vi "write_ini_SavedPos.vi"(8 "error in (no error)":errorcluster caption="错误输入（无错误）", 10 "file ref in":T1, 11 "MotorSystem 输入":refnum<class "MotorSystem.lvclass">) -> (0 "error out":errorcluster caption="错误输出", 2 "file ref out":T1, 3 "MotorSystem 输出":refnum<class "MotorSystem.lvclass">)   [LabVIEW 2016, in "MotionControl_UFO_3DOF.lvlib" / "MotorSystem.lvclass"]
uses:
  <userlib>/MotionControl_UFO_3DOF/MotorSystem/MotorSystem.lvclass
  <vilib>/Utility/config.llb/Config Data RefNum.ctl
  <userlib>/MotionControl_UFO_3DOF/MotorSystem/MotorSystem.lvclass/MotorSystem.ctl
  <vilib>/Utility/config.llb/Write Key (I32).vi
  <vilib>/Utility/config.llb/Write Key (String).vi
  <vilib>/Utility/config.llb/Write Key (Double).vi
  <vilib>/Utility/config.llb/NI_LVConfig.lvlib
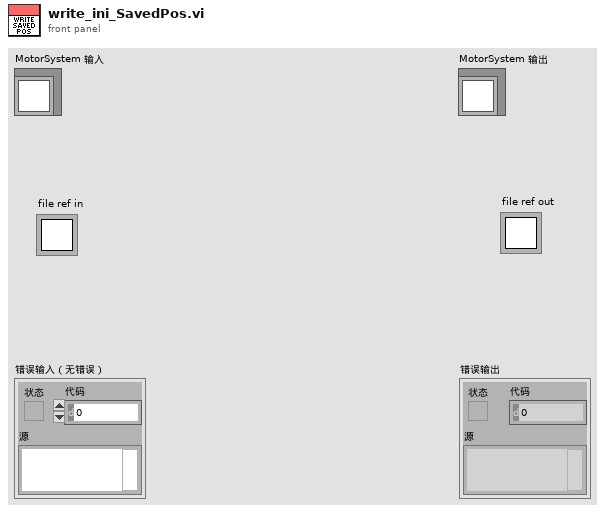
[diagram p1: front panel]
types:
  T1 = typedef "NI_LVConfig.lvlib/Config Data RefNum.ctl" = refnum<k1>
  T2 = typedef "MotionControl_UFO_3DOF.lvlib/MotorSystem.lvclass/SavedPosCluster.ctl" = cluster{"name":string, "command list":T3}
  T3 = typedef "MotionControl_UFO_3DOF.lvlib/MotorSystem.lvclass/CommandList.ctl" = cluster{"cmd":T4, "cmd info":T5[]}[]
  T4 = typedef "MotionControl_UFO_3DOF.lvlib/MotorSystem.lvclass/cmd_system.ctl" = enum16{"NONE", "MOVE_SYSTEM", "WAIT_UNTIL_MOVE_DONE", "EXIT", "WAIT_UNTIL_SELECTED_MOVE_DONE", "WAIT_A_TIME"}
  T5 = typedef "MotionControl_UFO_3DOF.lvlib/MotorSystem.lvclass/SavedDimensionCluster.ctl" = cluster{"dimension name":string, "pos":dbl, "unit mode":T6, "unit conversion ratio":dbl}
  T6 = typedef "MotionControl_UFO_3DOF.lvlib/OneMotion.lvclass/unit mode.ctl" = enum16{"motor (pulse)", "linear (mm) or radial (degree)"}
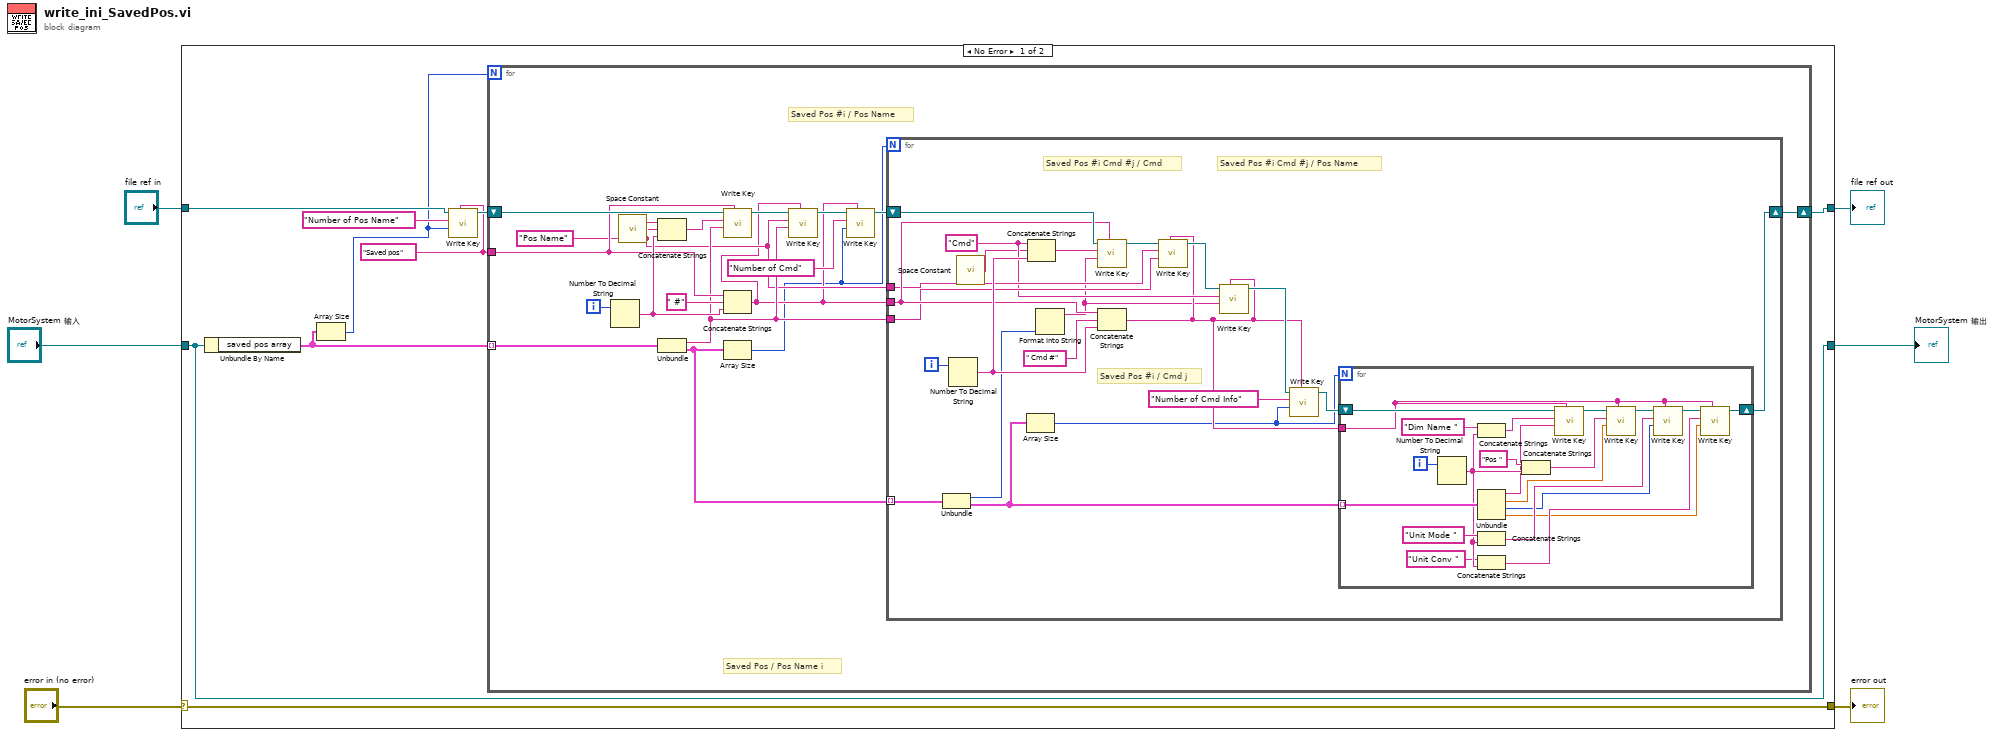
[diagram p0: block diagram]
diagram:
  n1 = case shown="No Error" "error in (no error)" {
    selector: "error in (no error)" -> [w15 w79]
    tunnel: [w15 w79] -> w5
    tunnel: [w14 w78] -> w3
    tunnel: "MotorSystem 输入" -> [w14 w78]
    tunnel: "file ref in" -> [w10 w77]
    tunnel: [w12 w77] -> w1
    frame No Error {
      w7 = "Saved pos"
      n2 = Unbundle By Name(w14) -> ("saved pos array"=w13:T2[])
      n3 = Array Size(array=w13) -> (size(s)=w8:i32)
      n4 = call-poly <vilib>:"Write Key.vi"("section"=w7, "value"=w8, "key"="Number of Pos Name", "refnum"=w10) -> ("refnum out"=w9:T1)  [unwired: 5 in, 2 out]
      n5 = for {
        N: w8 -> [_]
        tunnel: w13 -> [w30] mode=indexing
        shift-right: [w28] -> w12
        shift-left: w9 -> [w32]
        tunnel: w7 -> [w24]
        i -> [w31]
        w22 = "Pos Name"
        # "Saved Pos #i / Pos Name"
        # "Saved Pos / Pos Name i"
        n6 = Number To Decimal String(number=w31) -> (decimal integer string=w26:string)  [unwired: 1 in]
        n7 = call <vilib>:"Space Constant.vi"() -> ("String"=w21:string)
        n8 = Concatenate Strings(w22, w21, w26) -> (w33:string)
        n9 = Unbundle(w30) -> ("name"=w23:string, "command list"=w29:T3)
        n10 = call-poly <vilib>:"Write Key.vi"("section"=w24, "value"=w23, "key"=w33, "refnum"=w32) -> ("refnum out"=w25:T1)  [unwired: 5 in, 2 out]
        n11 = Concatenate Strings(w24, " #", w26) -> (w17:string)
        n12 = Array Size(array=w29) -> (size(s)=w16:i32)
        n13 = call-poly <vilib>:"Write Key.vi"("section"=w17, "value"=w23, "key"=w22, "refnum"=w25) -> ("refnum out"=w19:T1)  [unwired: 5 in, 2 out]
        n14 = call-poly <vilib>:"Write Key.vi"("section"=w17, "value"=w16, "key"="Number of Cmd", "refnum"=w19) -> ("refnum out"=w18:T1)  [unwired: 5 in, 2 out]
        n15 = for {
          N: w16 -> [_]
          tunnel: w29 -> [w54] mode=indexing
          tunnel: w17 -> [w48]
          shift-right: [w55] -> w28
          shift-left: w18 -> [w49]
          tunnel: w22 -> [w45]
          tunnel: w23 -> [w47]
          i -> [w53]
          w42 = "Cmd"
          # "Saved Pos #i Cmd #j / Cmd"
          # "Saved Pos #i Cmd #j / Pos Name"
          # "Saved Pos #i / Cmd j"
          n16 = Unbundle(w54) -> ("cmd"=w43:T4, "cmd info"=w36:T5[])
          n17 = Number To Decimal String(number=w53) -> (decimal integer string=w50:string)  [unwired: 1 in]
          n18 = call <vilib>:"Space Constant.vi"() -> ("String"=w41:string)
          n19 = Array Size(array=w36) -> (size(s)=w35:i32)
          n20 = Concatenate Strings(w42, w41, w50) -> (w52:string)
          n21 = Format Into String(w43) -> (resulting string=w34:string)  [unwired: 3 in, 1 out]
          n22 = call-poly <vilib>:"Write Key.vi"("section"=w48, "value"=w34, "key"=w52, "refnum"=w49) -> ("refnum out"=w46:T1)  [unwired: 5 in, 2 out]
          n23 = Concatenate Strings(w48, " Cmd #", w50) -> (w37:string)
          n24 = call-poly <vilib>:"Write Key.vi"("section"=w37, "value"=w47, "key"=w45, "refnum"=w46) -> ("refnum out"=w44:T1)  [unwired: 5 in, 2 out]
          n25 = call-poly <vilib>:"Write Key.vi"("section"=w37, "value"=w34, "key"=w42, "refnum"=w44) -> ("refnum out"=w39:T1)  [unwired: 5 in, 2 out]
          n26 = call-poly <vilib>:"Write Key.vi"("section"=w37, "value"=w35, "key"="Number of Cmd Info", "refnum"=w39) -> ("refnum out"=w38:T1)  [unwired: 5 in, 2 out]
          n27 = for {
            N: w35 -> [_]
            tunnel: w36 -> [w76] mode=indexing
            shift-right: [w61] -> w55
            shift-left: w38 -> [w73]
            tunnel: w37 -> [w60]
            i -> [w75]
            n28 = Number To Decimal String(number=w75) -> (decimal integer string=w67:string)  [unwired: 1 in]
            n29 = Concatenate Strings("Dim Name ", w67) -> (w56:string)
            n30 = Unbundle(w76) -> ("dimension name"=w57:string, "pos"=w69:dbl, "unit mode"=w59:T6, "unit conversion ratio"=w58:dbl)
            n31 = Concatenate Strings("Unit Mode ", w67) -> (w64:string)
            n32 = Concatenate Strings("Unit Conv ", w67) -> (w65:string)
            n33 = Concatenate Strings("Pos ", w67) -> (w71:string)
            n34 = call-poly <vilib>:"Write Key.vi"("section"=w60, "value"=w57, "key"=w56, "refnum"=w73) -> ("refnum out"=w70:T1)  [unwired: 5 in, 2 out]
            n35 = call-poly <vilib>:"Write Key.vi"("section"=w60, "value"=w69, "key"=w71, "refnum"=w70) -> ("refnum out"=w63:T1)  [unwired: 5 in, 2 out]
            n36 = call-poly <vilib>:"Write Key.vi"("section"=w60, "value"=w59, "key"=w64, "refnum"=w63) -> ("refnum out"=w62:T1)  [unwired: 5 in, 2 out]
            n37 = call-poly <vilib>:"Write Key.vi"("section"=w60, "value"=w58, "key"=w65, "refnum"=w62) -> ("refnum out"=w61:T1)  [unwired: 5 in, 2 out]
          }
        }
      }
    }
    frame Error {
    }
  }
  "error out" <- w5
  "MotorSystem 输出" <- w3
  "file ref out" <- w1
